vi "DMACalcs.vi"(8 "Number of Channels":u32=1, 9 "Number of Samples":u32, 11 "Rate (Hz)":dbl) -> (0 "Block Size":u32, 1 "Time to Acquire Block (ms)":i32, 3 "Host Buffer Size":u32)   [LabVIEW 2017, in "HostCode.lvlib"]
doc: "This VI performs calculations needed to set up and perform DMA transfers.\n\n<B>Inputs:</B>\n<B>Rate (Hz)</B> - Rate in Hz of the acquisition.\n<B>Number of Samples</B> - The number of samples of each channel to be taken per DMA read.\n<B>Number of Channels</B> - The number of channels being read.\n\n<B>Outputs:</B>\n<B>Time to Acquire Block (ms)</B> - Amount of time needed by the FPGA to acquire a block of data.\n<B>Host Buffer Size</B> - This value should be used to set the host buffer size. It is set to be three times the <B>Block Size</B>.\n<B>Block Size</B> - The amount of data to be read from the DMA buffer. This is calculated by multiplying the <B>Number of Samples</B> by the <B>Number of Channels</B>."
uses:
  HostCode.lvlib
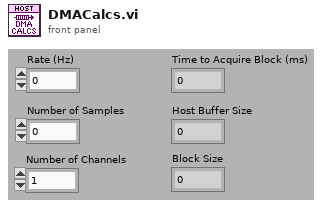
[diagram p1: front panel]
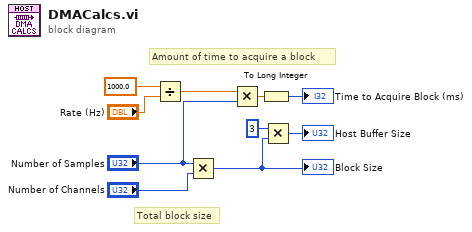
[diagram p0: block diagram]
diagram:
  # "Total block size"
  # "Amount of time to acquire a block"
  n1 = Divide(x=1000.0 ("y"), y="Rate (Hz)") -> (x/y=w1:dbl)
  n2 = Multiply(x="Number of Samples", y="Number of Channels") -> (x*y=w9:u32)
  "Block Size" <- w9
  n3 = Multiply(x=w1, y="Number of Samples") -> (x*y=w7:dbl)
  n4 = To Long Integer(number=w7) -> (32bit integer=→"Time to Acquire Block (ms)":i32)
  n5 = Multiply(x=u32 3, y=w9) -> (x*y=→"Host Buffer Size":u32)
